vi "GetMetadataCount.vi"(8 "error in (no error)":errorcluster, 11 "session id in":i32) -> (0 "error out":errorcluster, 2 "MetadataCount":i32, 3 "session id out":i32)   [LabVIEW 2017, in "libonnx_wrapper.lvlib"]
doc: "/**\n * @brief Получить количество метаданных модели\n * \n * ONNX модели могут содержать метаданные: версию, имя автора, описание и т.д.\n * \n * @param sessionId [IN] ID сессии\n * \n * @return int32: Количество пар ключ-значение\n * @return int32: 0 если сессия не найдена или метаданных нет\n */\nint GetMetadataCount(int sessionId);"
uses:
  libonnx_wrapper.lvlib
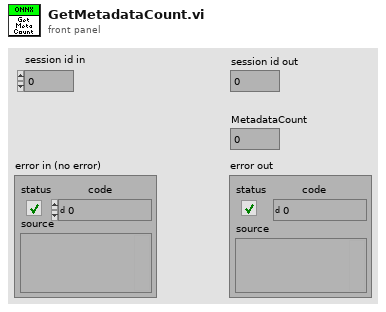
[diagram p1: front panel]
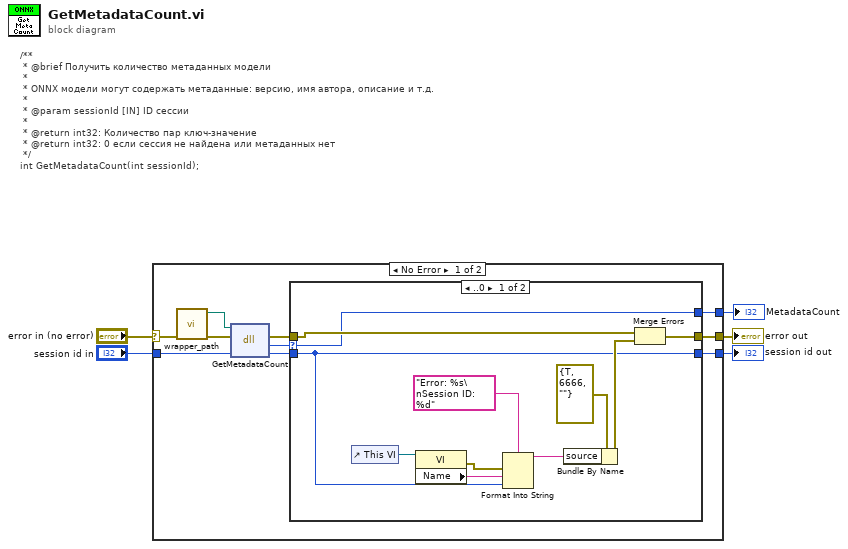
[diagram p0: block diagram]
diagram:
  # "/**\n * @brief Получить количество метаданных модели\n * \n * ONNX модели могут содержать метаданные: версию, имя автора, описание и т.д.\n * \n * @param sessionId [IN] ID сессии\n * \n * @return int32: Количество пар ключ-значение\n * @return int32: 0 если сессия не найдена или метаданных нет\n */\nint GetMetadataCount(int sessionId);"
  n1 = case shown="No Error" "error in (no error)" {
    selector: "error in (no error)" -> [w6 w31]
    tunnel: "session id in" -> [w13 w30]
    tunnel: [w9 w31] -> w4
    tunnel: [w8 _] -> w3
    tunnel: [w7 w30] -> w2
    frame No Error {
      n2 = call "wrapper_path.vi"("error in (no error)"=w6) -> ("error out"=w15:errorcluster, "wrapper path"=w14:path)  [unwired: 9 in]
      n3 = dll-call lib="home/ivan/LabVIEWData/ONNX/Test/libonnx_wrapper/unix64/libonnx_wrapper.so" fn="GetMetadataCount"(path in=w14, error in=w15, "sessionId"=w13) -> (error out=w12:errorcluster, "MetadataCount"=w11:i32, "sessionId"=w10:i32)  [unwired: 1 in, 1 out]
      n4 = case shown="..0" w11 {
        selector: w11 -> [w16 w27]
        tunnel: w12 -> [w17 w29]
        tunnel: [w18 w29] -> w9
        tunnel: w10 -> [w19 w28]
        tunnel: [w19 w28] -> w7
        tunnel: [w16 w27] -> w8
        frame ..0 {
          n5 = control-ref of="This VI"() -> (w23:refnum<vi>)
          n6 = property class="VI"(reference=w23) -> (error out=w20:errorcluster, "Name"=w22:string)  [unwired: 1 in, 1 out]
          n7 = Format Into String(format string="Error: %s\nSession ID: %d", error in=w20, w22, w19) -> (resulting string=w24:string)  [unwired: 1 in, 1 out]
          n8 = Bundle By Name(cluster=errorcluster {"status"=TRUE, "code"=6666, "source"=""} ("error out"), "source"=w24) -> (w25:errorcluster)
          n9 = Merge Errors(w17, w25) -> (w18:errorcluster)
        }
        frame 1.. {
        }
      }
    }
    frame Error {
    }
  }
  "error out" <- w4
  "session id out" <- w2
  "MetadataCount" <- w3
